vi "MasterAccelerometerSampleCameraRotator.vi"   [LabVIEW 2018]
uses:
  <vilib>/rvi/Emulation/niFpgaGetClockAttributes.vi
  <vilib>/rvi/Emulation/niFpgaSctlEmulationGetInTimedLoop.vi
  <vilib>/rvi/Emulation/niFpgaEmulationReportErrorSimple.vi
  <vilib>/rvi/eio/common/nirviEmuTemplateMethod_errors.vi
  <vilib>/rvi/Emulation/niFpgaEmulationIsFPGAContextNoSignature.vi
  <vilib>/rvi/DataTransferAndStorage/Container/Common/niFpgaContainerGetUniqueNameForEmu.vi
  <vilib>/rvi/Memory/Memory_Emulation/niFpgaMemoryEmulationCacheClearOnFirstRun.vi
  <vilib>/rvi/Memory/Memory_Emulation/nirvimemoryEmulationManagerCache_MakeExclusive.vi
  <vilib>/rvi/Memory/Memory_Emulation/niFpgaMemoryEmulationValidateCache.vi
  <vilib>/rvi/Memory/Memory_Emulation/nirvimemoryEmulationManagerCache_InsertValue.vi
  <vilib>/Utility/error.llb/Clear Errors.vi
  <vilib>/rvi/Memory/Memory_Emulation/nirvimemoryEmulationManagerCache_ReleaseExclusive.vi
  <vilib>/rvi/Memory/Memory_Emulation/nirvimemoryEmulationManagerCache_GetValue.vi
  <vilib>/rvi/Memory/Memory_Emulation/nirvimemoryEmulationManagerCache_SetValue.vi
  <vilib>/rvi/Emulation/niFpgaProcessEmulError.vi
  <vilib>/rvi/errors/niFpgaSetErrorForExecOnDevCompSimple.vi
  <vilib>/rvi/eio/common/nirviEmuReportErrorAndStop.vi
  <vilib>/rvi/FIFO/Fifo_Resource/nirvififoEmulationSetSize.vi
  <vilib>/rvi/FIFO/Fifo_Resource/nirviFifoEmulationQueueMgr.vi
  <instcachedir>/0/nirviFifoEmulationQueueMgr_E5CAEC123FF24DC58D834DCA3CDAA9B5.lvgen/nirviFifoEmulationQueueMgr_E5CAEC123FF24DC58D834DCA3CDAA9B5_017.vi
  <vilib>/rvi/FIFO/Fifo_Resource/nirvififoEmulationDetermineInputValidOut.vi
  <vilib>/rvi/FIFO/Fifo_Resource/nirvififoEmulationCreateLock.vi
  <vilib>/rvi/FIFO/Fifo_Resource/nirvififoEmulationObtainLock.vi
  <vilib>/rvi/FIFO/Fifo_Resource/nirvififoEmulationReleaseLock.vi
  <vilib>/rvi/occurrence/nirviWaitOnOccurrenceBase.vi
  <vilib>/rvi/errors/nirviReportUnexpectedCaseInternalError.vi
  <vilib>/rvi/errors/nirviReportUnexpectedCaseInternalError (U32).vi
  <instcachedir>/0/nirviFifoEmulationQueueMgr_E5CAEC123FF24DC58D834DCA3CDAA9B5.lvgen/nirviFifoEmulationQueueMgr_E5CAEC123FF24DC58D834DCA3CDAA9B5_023.vi
  <vilib>/rvi/Emulation/niFpgaCriticalErrorInLSC.vi
  <vilib>/eio/EIONode/EIONode.xnode
  <vilib>/rvi/DataTransferAndStorage/Container/XNode/niFpgaContainer.xnode
  <vilib>/rvi/DataTransferAndStorage/Register/Emulation/niFpgaRegisterEmulation.vi
  <vilib>/rvi/FIFO/Fifo_Resource/nirvififoEmulationWrite.vi
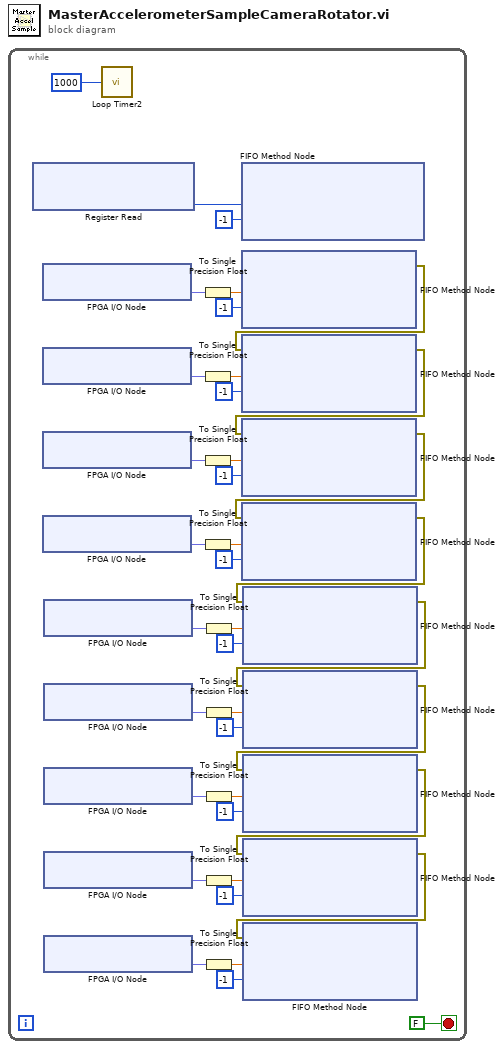
[diagram p0: block diagram]
diagram:
  n1 = while {
    stop <- FALSE stop-if-true
    n2 = xnode ("Register Read")() -> ("Data"=w2:u64)  [unwired: 1 in, 1 out]
    n3 = xnode "FPGA I/O Node"() -> ("Accelerometer1/AI0"=w37:fxp<+/-,24,7>)  [unwired: 1 in, 1 out]
    n4 = xnode "FPGA I/O Node"() -> ("Accelerometer1/AI1"=w32:fxp<+/-,24,7>)  [unwired: 1 in, 1 out]
    n5 = xnode "FPGA I/O Node"() -> ("Accelerometer1/AI2"=w24:fxp<+/-,24,7>)  [unwired: 1 in, 1 out]
    n6 = xnode "FPGA I/O Node"() -> ("Accelerometer2/AI0"=w29:fxp<+/-,24,7>)  [unwired: 1 in, 1 out]
    n7 = xnode "FPGA I/O Node"() -> ("Accelerometer2/AI1"=w8:fxp<+/-,24,7>)  [unwired: 1 in, 1 out]
    n8 = xnode "FPGA I/O Node"() -> ("Accelerometer2/AI2"=w13:fxp<+/-,24,7>)  [unwired: 1 in, 1 out]
    n9 = xnode "FPGA I/O Node"() -> ("Accelerometer3/AI0"=w21:fxp<+/-,24,7>)  [unwired: 1 in, 1 out]
    n10 = xnode "FPGA I/O Node"() -> ("Accelerometer3/AI1"=w16:fxp<+/-,24,7>)  [unwired: 1 in, 1 out]
    n11 = xnode "FPGA I/O Node"() -> ("Accelerometer3/AI2"=w4:fxp<+/-,24,7>)  [unwired: 1 in, 1 out]
    n12 = call "Loop Timer2"("Count(uSec)"=u32 1000 ("Data")) -> ()  [unwired: 1 out]
    n13 = To Single Precision Float(number=w37) -> (single precision float=w36:sgl)
    n14 = To Single Precision Float(number=w32) -> (single precision float=w33:sgl)
    n15 = To Single Precision Float(number=w24) -> (single precision float=w25:sgl)
    n16 = To Single Precision Float(number=w29) -> (single precision float=w28:sgl)
    n17 = To Single Precision Float(number=w8) -> (single precision float=w9:sgl)
    n18 = To Single Precision Float(number=w13) -> (single precision float=w12:sgl)
    n19 = To Single Precision Float(number=w21) -> (single precision float=w20:sgl)
    n20 = To Single Precision Float(number=w16) -> (single precision float=w17:sgl)
    n21 = To Single Precision Float(number=w4) -> (single precision float=w5:sgl)
    n22 = xnode ("FIFO Method Node")("Element"=w2, "Timeout"=-1) -> ()  [unwired: 1 in, 2 out]
    n23 = xnode ("FIFO Method Node")("Element"=w36, "Timeout"=-1) -> ("error out"=w31:errorcluster)  [unwired: 2 in, 2 out]
    n24 = xnode ("FIFO Method Node")("Element"=w33, "Timeout"=-1, "error in (no error)"=w31) -> ("error out"=w23:errorcluster)  [unwired: 1 in, 2 out]
    n25 = xnode ("FIFO Method Node")("Element"=w25, "Timeout"=-1, "error in (no error)"=w23) -> ("error out"=w30:errorcluster)  [unwired: 1 in, 2 out]
    n26 = xnode ("FIFO Method Node")("Element"=w28, "Timeout"=-1, "error in (no error)"=w30) -> ("error out"=w7:errorcluster)  [unwired: 1 in, 2 out]
    n27 = xnode ("FIFO Method Node")("Element"=w9, "Timeout"=-1, "error in (no error)"=w7) -> ("error out"=w14:errorcluster)  [unwired: 1 in, 2 out]
    n28 = xnode ("FIFO Method Node")("Element"=w12, "Timeout"=-1, "error in (no error)"=w14) -> ("error out"=w22:errorcluster)  [unwired: 1 in, 2 out]
    n29 = xnode ("FIFO Method Node")("Element"=w20, "Timeout"=-1, "error in (no error)"=w22) -> ("error out"=w15:errorcluster)  [unwired: 1 in, 2 out]
    n30 = xnode ("FIFO Method Node")("Element"=w17, "Timeout"=-1, "error in (no error)"=w15) -> ("error out"=w3:errorcluster)  [unwired: 1 in, 2 out]
    n31 = xnode ("FIFO Method Node")("Element"=w5, "Timeout"=-1, "error in (no error)"=w3) -> ()  [unwired: 1 in, 3 out]
  }
